vi "全局步骤树形列表相关.vi"() -> ()   [LabVIEW 2016]
panel:
  out "跳转次数变量":i32=2
  in  "数据数组":string[][](array[string])
  in  "数据存储时间间隔（分钟）":dbl format="%#g"
  out "当前步骤":i32
  out "多位阀的位置":string
  out "T(cool)℃":string
  out "P（eq)mv":string
  out "R(Gas)mv":string
  out "F(Flow)ml/min":string
  out "x*y":i32
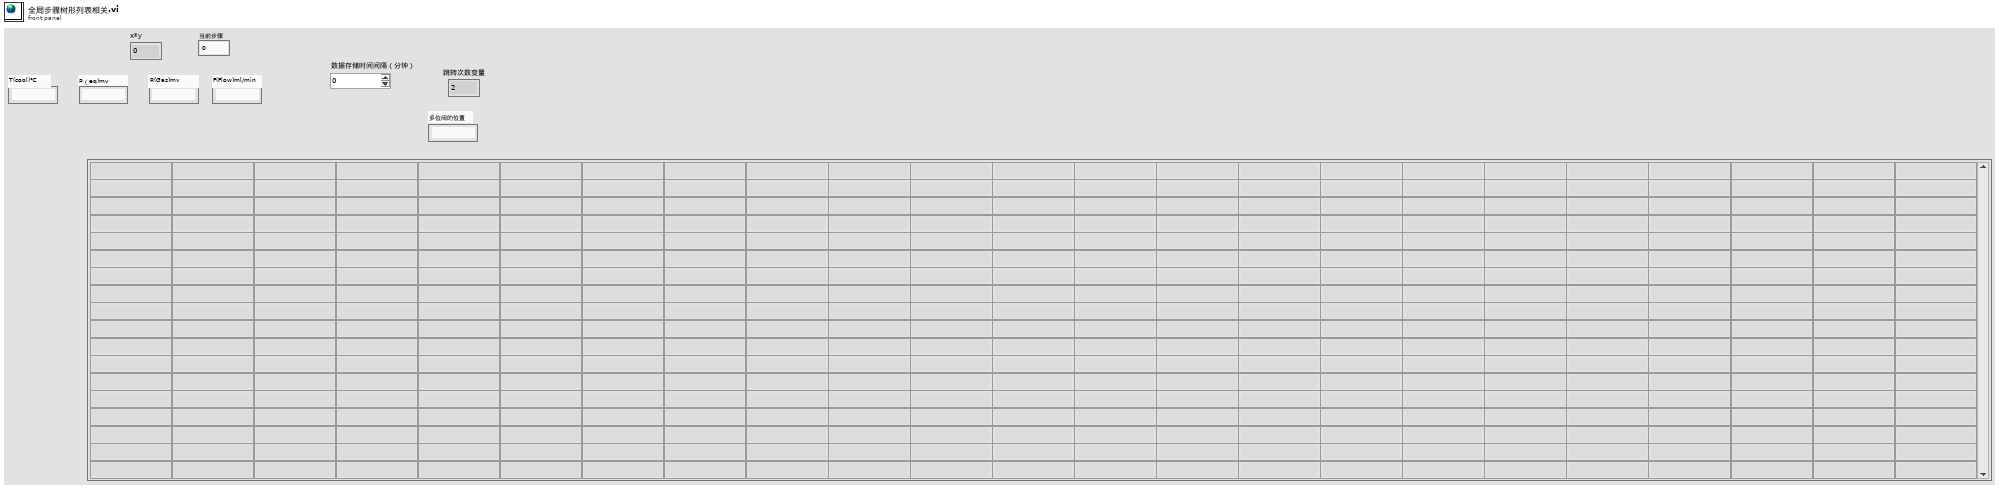
[diagram p1: front panel]
diagram:
